vi "getData.vi"(8 "error in (no error)":errorcluster, 11 "reference in":refnum<class "Notification Controller.lvclass">) -> (0 "error out":errorcluster, 2 "data":string[][][](array[string]), 3 "reference out":refnum<class "Notification Controller.lvclass">)   [LabVIEW 2015, in "Notification Controller.lvclass"]
uses:
  Notification Controller.lvclass
  APP/excelFile_class/fileType.ctl
  File Controller_llb/File Controller.lvclass
  APP/excelFile_class/excelFile.lvclass
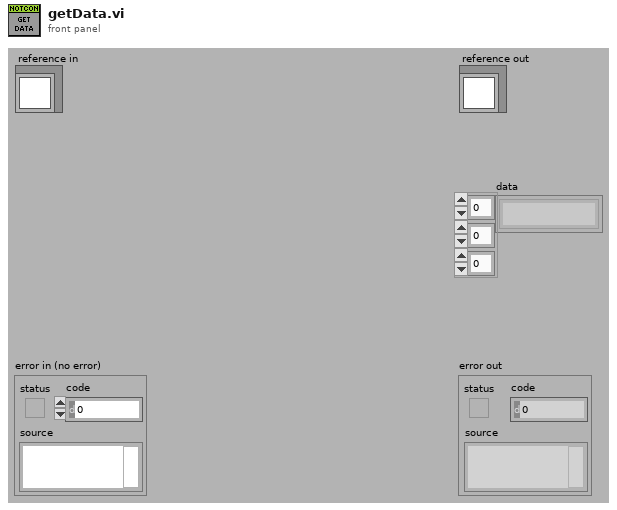
[diagram p1: front panel]
types:
  T1 = typedef "excelFile.lvclass/fileType.ctl" = enum16{"devices", "items", "partsTracking", "TSR"}
  T2 = typedef "Notification Controller.lvclass/ObjectAttributesRef.ctl" = refnum<data-value>
  T3 = typedef "Notification Controller.lvclass/ObjectAttributes.ctl" = cluster{"MyAttribute":dbl, "items_data":string[][][], "items_notification_refs":refnum<class "itemsNotification.lvclass">[], "notifications_data_items":string[][], "items_nots?":bool, "devices_controller_ref":refnum<class "Devices Controller.lvclass">, "onlineUpdate":timestamp, "notController?":bool, "tracking_notification_ref":refnum<class "trackingNotification.lvclass">, "notifications_data_tracking":string[][], "tracking_parts_data":string[][], "tracking_nots?":bool, "index_tracking_not":i32[], "file_controller_ref":refnum<class "File Controller.lvclass">}
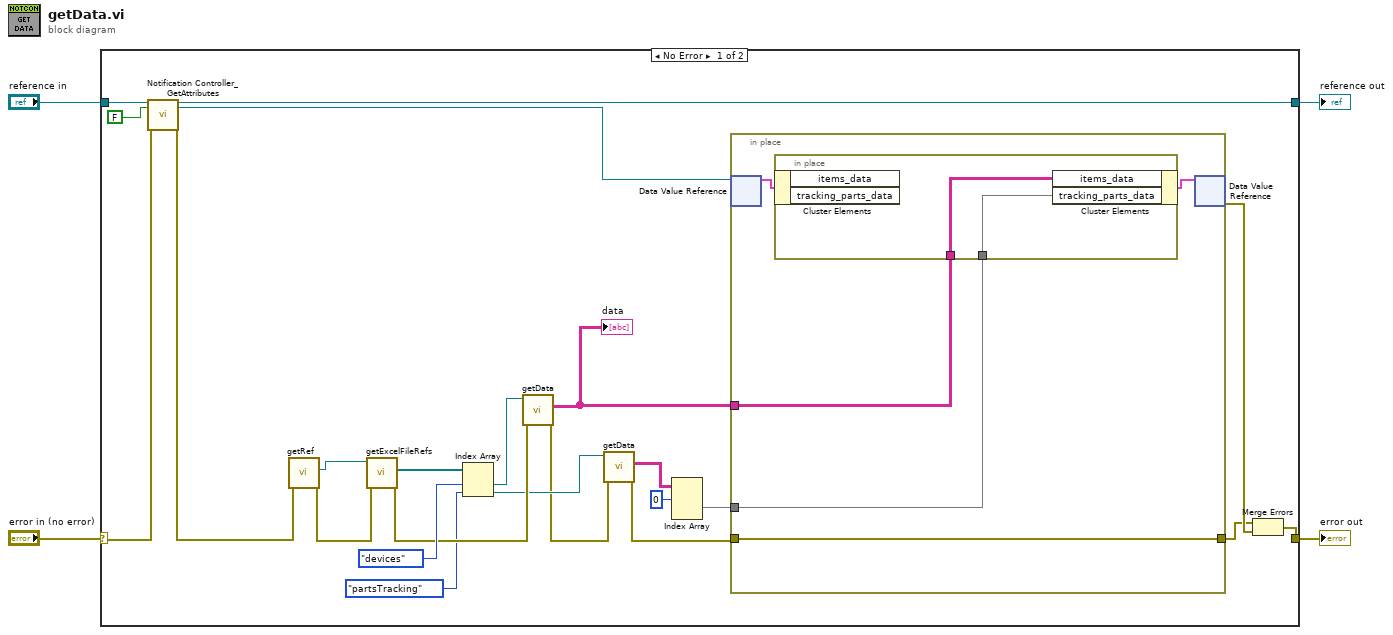
[diagram p0: block diagram]
diagram:
  n1 = case shown="No Error" "error in (no error)" {
    selector: "error in (no error)" -> [w22 w36]
    tunnel: [w27 w36] -> w3
    tunnel: [w21 w35] -> w1
    tunnel: "reference in" -> [w24 w35]
    frame No Error {
      n2 = call "Notification Controller_GetAttributes.vi"("reference in"=w24, "return data? (T)"=FALSE, "error in (no error)"=w22) -> ("reference out"=w21:refnum<class "Notification Controller.lvclass">, "attributes ref"=w20:T2, "error out"=w13:errorcluster)  [unwired: 13 in, 1 out]
      n3 = call "getRef.vi"("error in (no error)"=w13) -> ("error out"=w18:errorcluster, "File Controller_ref"=w19:refnum<class "File Controller.lvclass">)  [unwired: 9 in]
      n4 = call "getExcelFileRefs.vi"("error in (no error)"=w18, "reference in"=w19) -> ("error out"=w15:errorcluster, "excelFile_refs"=w17:refnum<class "excelFile.lvclass">[])  [unwired: 7 in, 1 out]
      n5 = Index Array(array=w17, index #1=fileType."devices" ("fileType"), index #2=fileType."partsTracking" ("fileType")) -> (element #1=w14:refnum<class "excelFile.lvclass">, element #2=w10:refnum<class "excelFile.lvclass">)
      n6 = call "getData.vi"("error in (no error)"=w15, "reference in"=w14) -> ("error out"=w9:errorcluster, "data"=w12:string[][][])  [unwired: 7 in, 1 out]
      "data" <- w12
      n7 = call "getData.vi"("error in (no error)"=w9, "reference in"=w10) -> ("error out"=w8:errorcluster, "data"=w7:string[][][])  [unwired: 7 in, 1 out]
      n8 = Index Array(array=w7, index (dim 0)=0 ("index (page)")) -> (element=w5:string[][])  [unwired: 2 in]
      n9 = in-place {
        in-place-border: w8 -> [w30]
        in-place-border: [w30] -> w25
        in-place-border: w12 -> [w29]
        in-place-border: w5 -> [w28]
        n10 = in-place-dvr #1(w20) -> (w31:T3)  [unwired: 1 out]
        n11 = in-place {
          in-place-border: w29 -> [w34]
          in-place-border: w28 -> [w33]
          n12 = in-place-cluster #2(w31) -> ()  [unwired: 2 out]
          n13 = in-place-cluster #2("items_data"=w34, "tracking_parts_data"=w33) -> (w32:T3)
        }
        n14 = in-place-dvr #1(w32) -> (w26:errorcluster)  [unwired: 1 out]
      }
      n15 = Merge Errors(w25, w26) -> (w27:errorcluster)
    }
    frame Error {
    }
  }
  "error out" <- w3
  "reference out" <- w1
